vi "ABB Test Bearing run.vi"() -> ()   [LabVIEW 2017]
uses:
  Temp error msg.ctl
  Video Display Buttons.ctl
  ABB global.vi
panel:
  in  "Video Displays":T1
  in  "Temp error":T2="Error: Temperature measurement "
  out "Primary coolant":u16(ring) items=["Oil", "Water", "Natural"]
  in  "Start":bool
  out "Additional Temperatures":string[][](table)
  in  "Stabilitymessg":string="Thermal Stability reached"
  out "Time to Next reading":dbl(slide) scale=0.0..2.0 scale format="%#.1f"
  out "Start Time":dbl
  out "Temperatures":string[][](table)
  out "Readings":string[][](table)
  out "saved Readings":dbl[][](array[numeric])
  out "Serial number":string
  out "W.O number":string
  out "Norma 5000 Error":string
  in  "Record":bool
  out "Reading table":string[][](table)
  in  "View":enum16{"Graph", "Readings"}(ring)
  out "Number readings":i32
  out "Status":enum16{"Stopped", "Running", "Finished"}(ring)
  out "Timedate":string
  in  "End test":bool
  in  "Read Mode":enum16{"Auto", "Manual"}(ring)
  in  "Exit":bool
  out "Temperature Trend":cluster{dbl[], "Best Linear Fit":dbl[]}[](graph)
  # "Bearing Run"
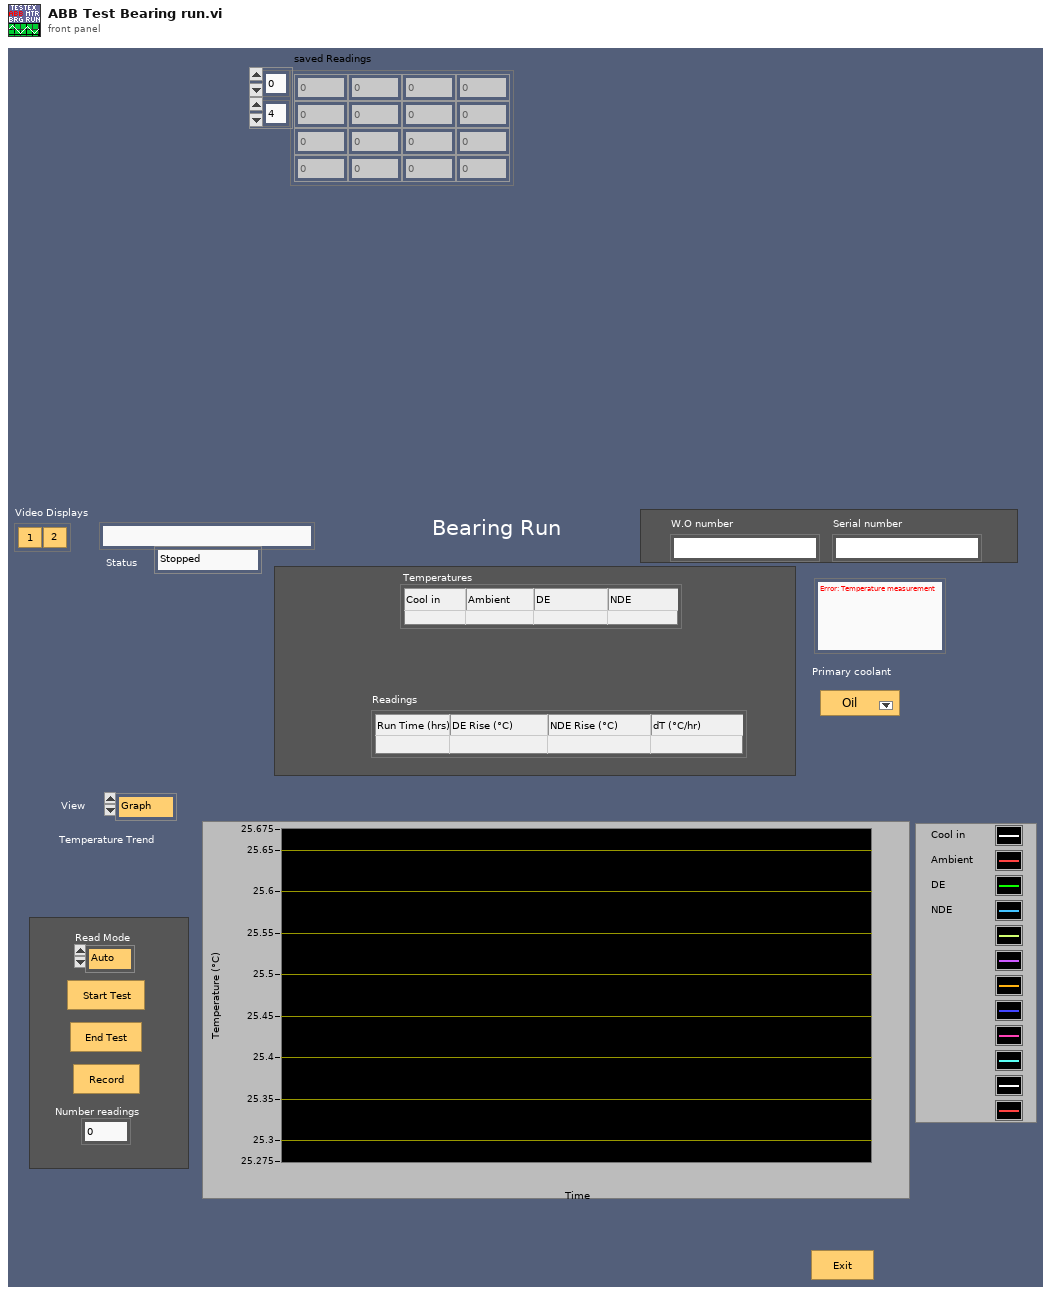
[diagram p1: front panel]
types:
  T1 = typedef "Video Display Buttons.ctl" = cluster{"1":bool, "1 2":bool}
  T2 = typedef "Temp error msg.ctl" = string
  T3 = enum16{"None", "Cool in", "Cool Out", "Wdg Temp", "Ambient", "DE", "NDE", "Aux coolant"}
  T4 = cluster{"VT Primary":dbl, "VT Secondary":dbl, "CT  Primary":dbl, "CT Secondary":dbl, "Current Shunt":enum16{"Internal", "External"}, "Avg interval":dbl}
  T5 = cluster{"VT Primary":dbl, "VT Secondary":dbl, "CT  Primary":dbl, "CT Secondary":dbl, "Current Shunt":enum16{"Internal", "External"}, "Averaging interval (secs)":dbl}
  T6 = cluster{"Visa sesssion":refnum<visa-resource-name>, "error":errorcluster}
  T7 = cluster{"Simulate Norma":bool, "Norma 5000 Address":u8, "WebDaq IP Address":string, "Simulate cDAQ":bool}
  T8 = cluster{"Thermal Stability (%)":dbl, "Reading interval (mins)":dbl}
  T9 = cluster{"String":string, "String":string, "String":string, "String":string}
  T10 = cluster{"String":dbl, "String":dbl, "String":dbl, "String":dbl}
  T11 = cluster{"temp. alloc":i32[], "category":i32[], "Category names":string[], "Category none names":string[]}
  T12 = cluster{"V":dbl, "A":dbl, "W":dbl, "VA":dbl, "VAr":dbl, "Pf":dbl}
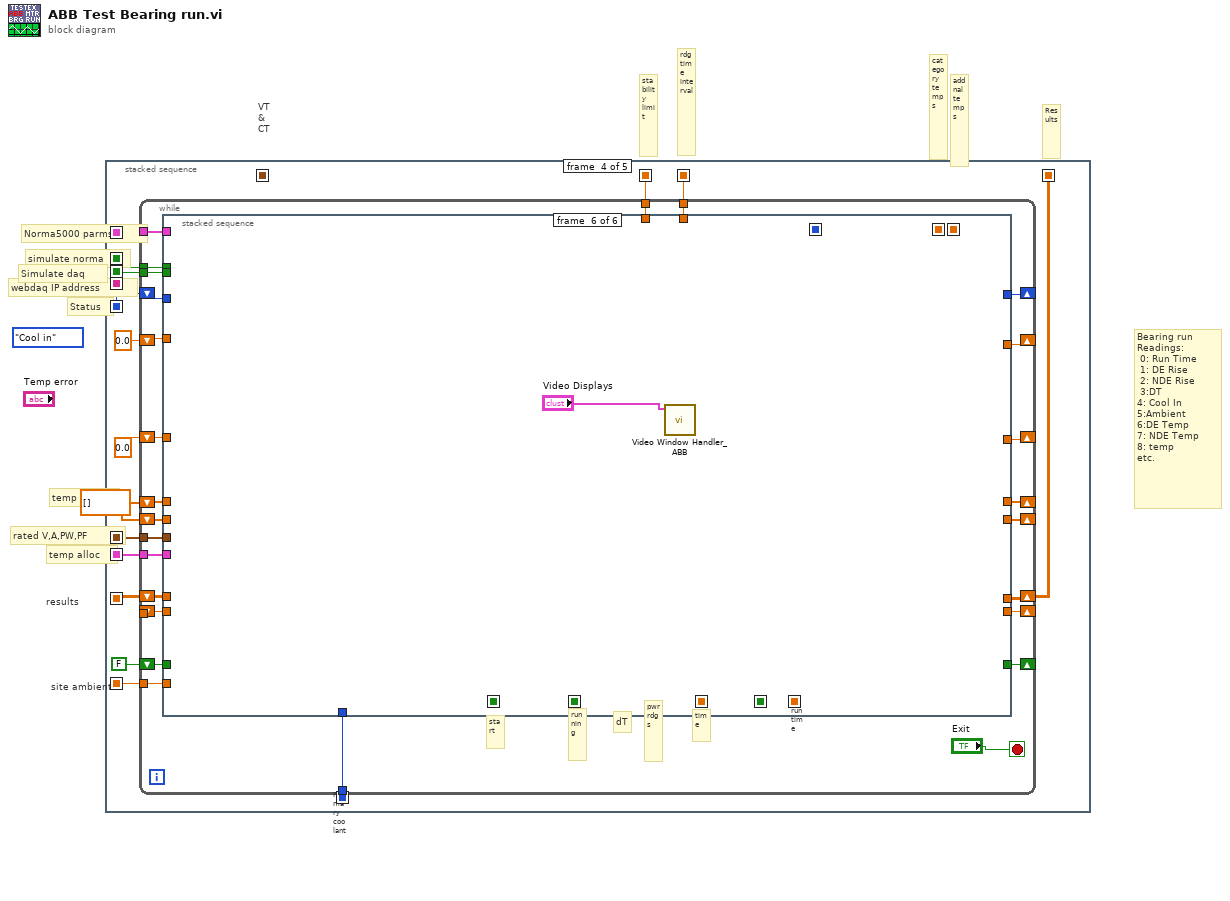
[diagram p0: block diagram]
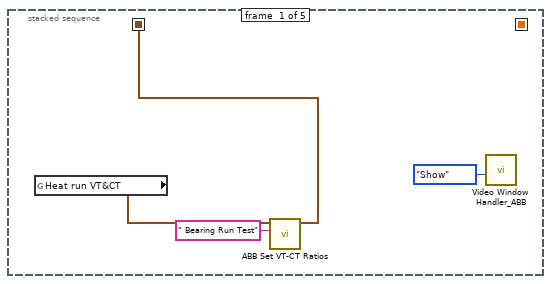
[diagram p2: hidden frame]
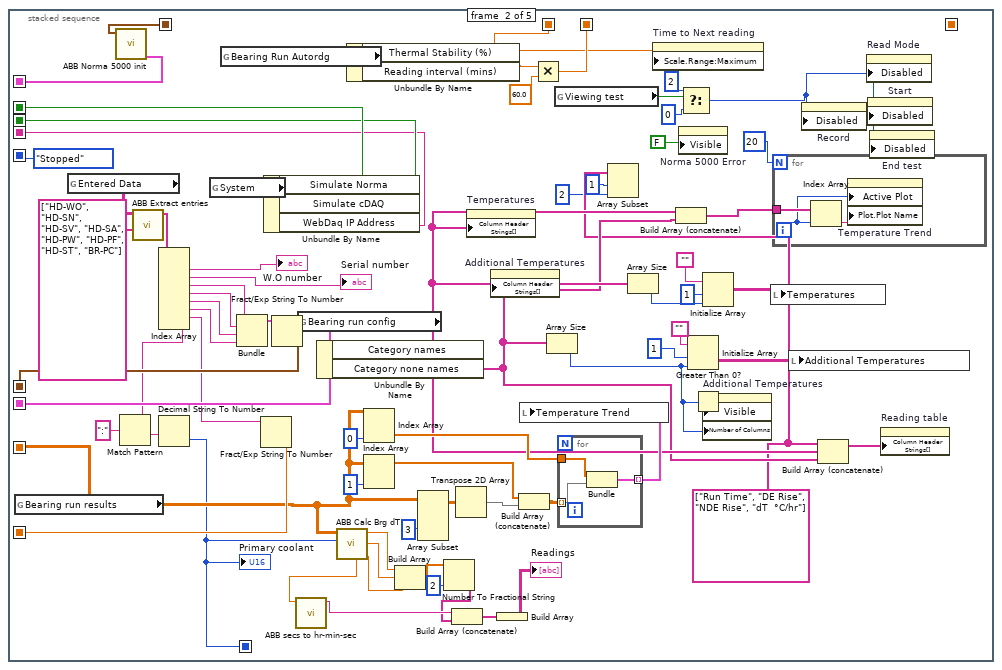
[diagram p3: hidden frame]
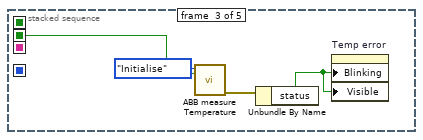
[diagram p4: hidden frame]
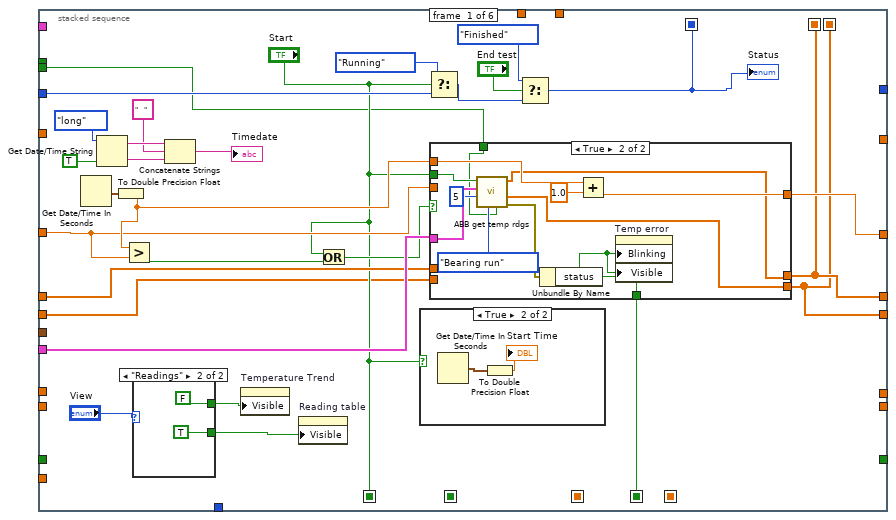
[diagram p5: hidden frame]
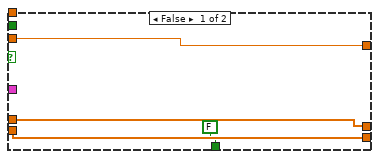
[diagram p7: hidden frame]
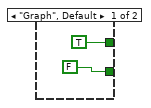
[diagram p8: hidden frame]
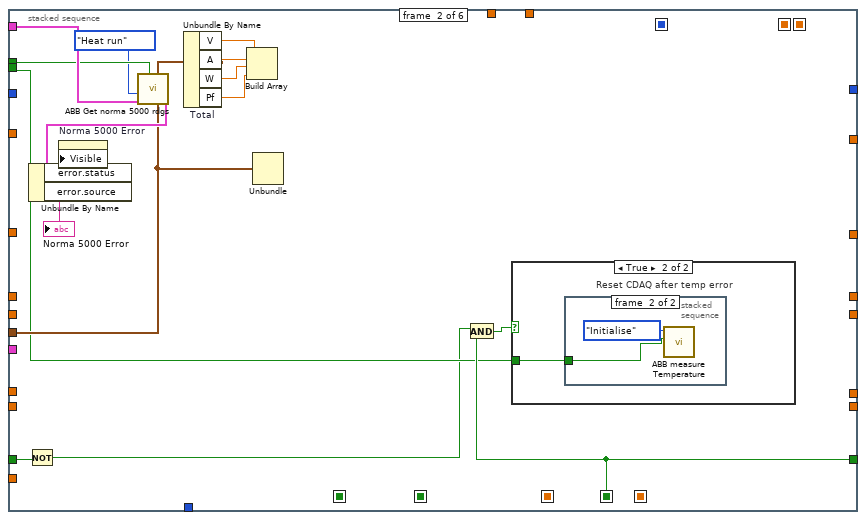
[diagram p9: hidden frame]
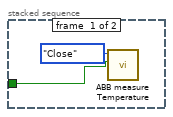
[diagram p11: hidden frame]
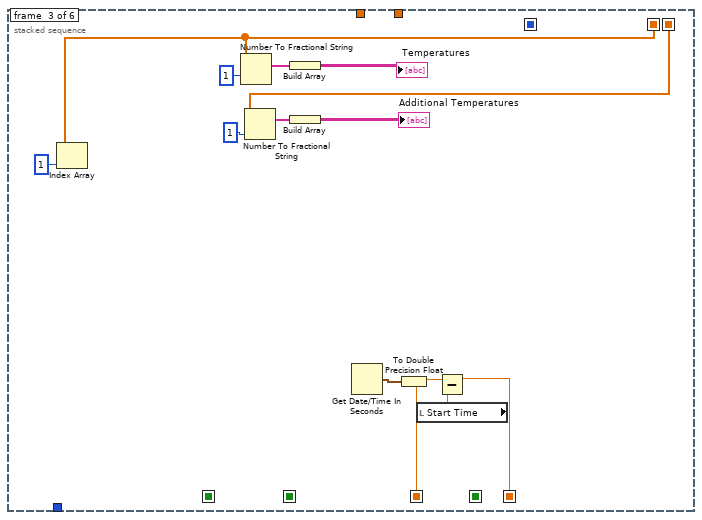
[diagram p12: hidden frame]
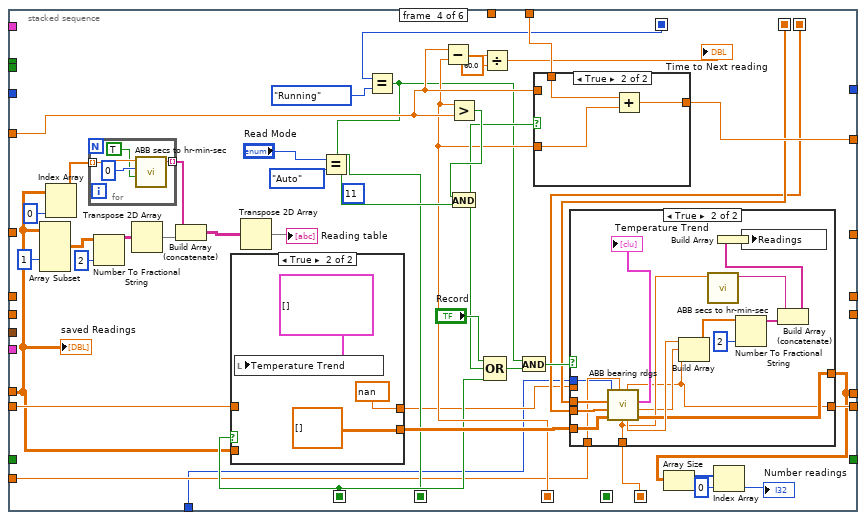
[diagram p13: hidden frame]
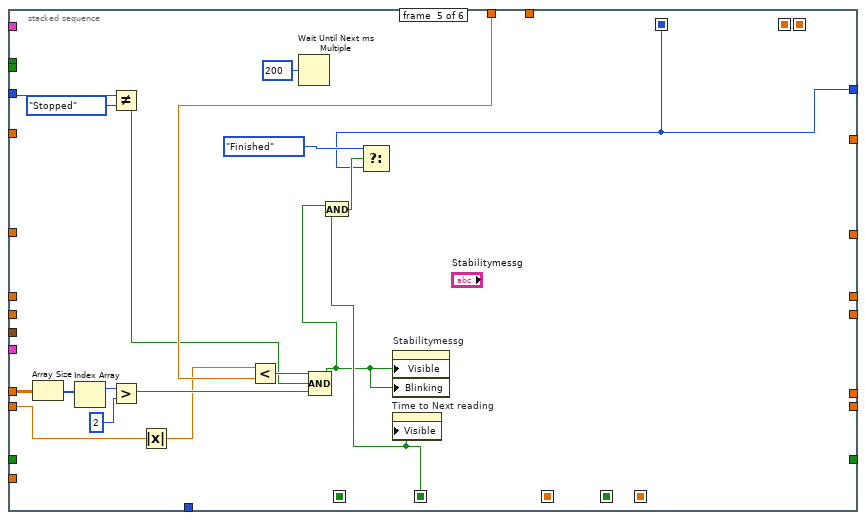
[diagram p17: hidden frame]
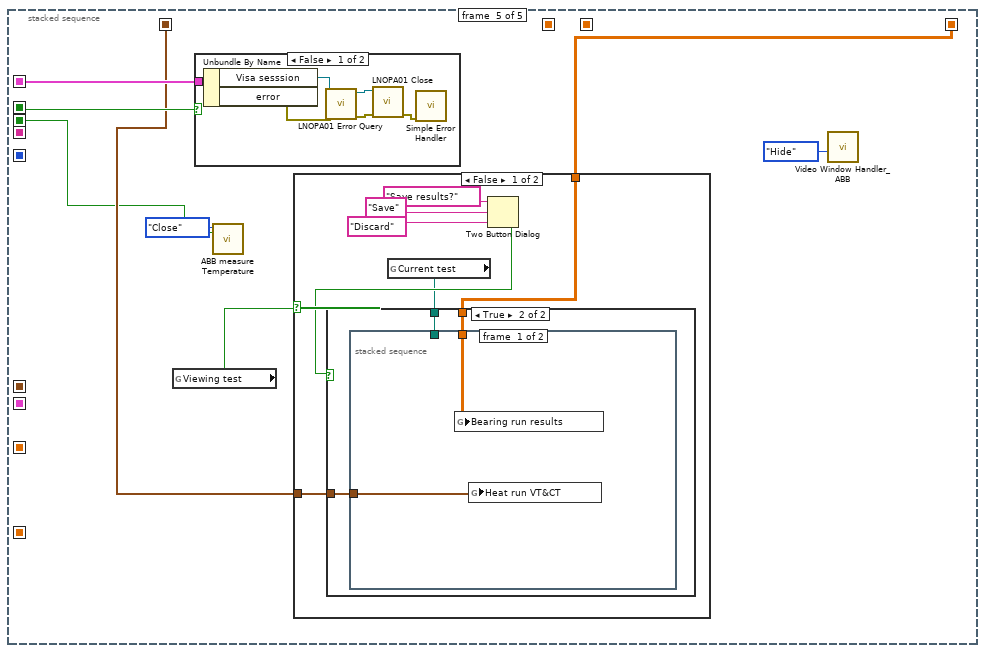
[diagram p18: hidden frame]
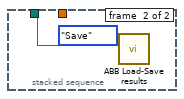
[diagram p20: hidden frame]
diagram:
  (unwired) T3."Cool in" ("Reading Category")
  # "Primary coolant"
  # "site ambient"
  # "results"
  # "VT & CT"
  # "webdaq IP address"
  # "Simulate daq"
  # "addnal temps"
  # "category temps"
  # "stability limit"
  # "Results"
  # "rdg time interval"
  # "Bearing run Readings:\n 0: Run Time\n 1: DE Rise\n 2: NDE Rise\n 3:DT\n4: Cool In\n5:Ambient\n6:DE Temp\n7: NDE Temp\n8: temp\netc."
  # "temp rdgs"
  # "temp alloc"
  # "rated V,A,PW,PF"
  # "simulate norma"
  # "Norma5000 parms"
  # "Status"
  n1 = stacked-sequence {
    seq-local: [_ enum16{"Stopped", "Running", "Finished"}."Stopped" ("Status") _ _ _] -> [_ _ _ w102 _]
    seq-local: [_ w75 _ _ _] -> [_ _ _ w101 w316]
    seq-local: [_ w72 _ _ _] -> [_ _ _ w100 w315]
    seq-local: [_ w71 _ _ _] -> [_ _ _ w99 _]
    seq-local: [_ w19 _ _ _] -> [_ _ _ w98 _]
    seq-local: [_ w35 _ _ _] -> [_ _ _ w97 _]
    seq-local: [_ w58 _ _ _] -> [_ _ _ w96 _]
    seq-local: [_ _ _ w94 _] -> [_ _ _ _ w313]
    seq-local: [_ w48 _ _ _] -> [_ _ _ w93 _]
    seq-local: [_ w32 _ _ _] -> [_ _ w86 w90 w310]
    seq-local: [_ w31 _ _ _] -> [_ _ _ _ _]
    seq-local: [w2 _ _ _ _] -> [_ w25 _ _ w312]
    seq-local: [_ w23 _ _ _] -> [_ _ _ w89 _]
    seq-local: [_ w18 _ _ _] -> [_ _ _ w88 _]
    frame #0 {
      n2 = global read "ABB global.vi" "Heat run VT&CT"() -> (w3:T4)
      n3 = call "ABB Set VT-CT Ratios.vi"("Test name"=" Bearing Run Test", "VT and CT Ratios"=w3) -> ("VT and CT Ratios out"=w2:T5)  [unwired: 9 in]
      n4 = call "Video Window Handler_ABB.vi"("Action"=enum16{"Show", "Hide", "Exit"}."Show") -> ()  [unwired: 11 in]
    }
    frame #1 {
      w7 = string[] ["Run Time", "DE Rise", "NDE Rise", "dT  °C/hr"]
      n5 = global read "ABB global.vi" "Bearing run results"() -> (w19:dbl[][])
      n6 = global read "ABB global.vi" "Entered Data"() -> (w55:string[][])
      n7 = call "ABB Norma 5000 init.vi"("VT and CT Ratios"=w25) -> ("norma 5000 parms out"=w75:T6)  [unwired: 10 in]
      n8 = call "ABB Extract entries.vi"("Entry IDs"=string[] ["HD-WO", "HD-SN", "HD-SV", "HD-SA", "HD-PW", "HD-PF", "HD-ST", "BR-PC"], "Entry table in"=w55) -> ("Selected Entries"=w53:string[])  [unwired: 9 in]
      n9 = Index Array(array=w53) -> (element #1=→"W.O number":string, element #2=→"Serial number":string, element #3=w50:string, element #4=w37:string, element #5=w36:string, element #6=w38:string, element #7=w24:string, element #8=w22:string)  [unwired: 8 in]
      n10 = Match Pattern(string=w22, regular expression=":") -> (after substring=w20:string)  [unwired: 1 in, 3 out]
      n11 = Decimal String To Number(string=w20) -> (number=w18:i32)  [unwired: 2 in, 1 out]
      "Primary coolant" <- w18
      n12 = global read "ABB global.vi" "System"() -> (w74:T7)
      n13 = global read "ABB global.vi" "Bearing Run Autordg"() -> (w70:T8)
      n14 = Bundle("String"=w50, "String"=w37, "String"=w36, "String"=w38) -> (w49:T9)  [unwired: 1 in]
      n15 = Fract/Exp String To Number(string=w24) -> (number=w23:dbl)  [unwired: 3 in, 1 out]
      n16 = Unbundle By Name(w74) -> ("Simulate Norma"=w72:bool, "Simulate cDAQ"=w32:bool, "WebDaq IP Address"=w31:string)
      n17 = Fract/Exp String To Number(string=w49) -> (number=w71:T10)  [unwired: 3 in, 1 out]
      n18 = global read "ABB global.vi" "Bearing run config"() -> (w35:T11)
      n19 = Unbundle By Name(w35) -> ("Category names"=w34:string[], "Category none names"=w29:string[])
      n20 = call "ABB Calc Brg dT.vi"("Primary coolant"=w18, "Readings in"=w19) -> ("dT (deg/hr)"=w13:dbl, "NDE rise"=w14:dbl, "DE rise"=w15:dbl, "run time"=w17:dbl)  [unwired: 5 in, 1 out]
      n21 = call "ABB secs to hr-min-sec.vi"("Seconds"=w17) -> ("hr:min:secs"=w16:string)  [unwired: 10 in]
      n22 = Unbundle By Name(w70) -> ("Thermal Stability (%)"=w48:dbl, "Reading interval (mins)"=w57:dbl)
      n23 = Index Array(array=w19, index (col)=0 ("disabled index (col)")) -> (element=w63:dbl[])  [unwired: 1 in]
      n24 = Index Array(array=w19, index (col)=1 ("disabled index (col)")) -> (element=w26:dbl[])  [unwired: 1 in]
      n25 = Build Array(w15, w14, w13) -> (w12:dbl[])
      n26 = Array Subset(array=w19, index (col)=3 ("index")) -> (w61:dbl[][])  [unwired: 3 in]
      n27 = Number To Fractional String(number=w12, precision (6)=i16 2) -> (F-format string=w10:string[])  [unwired: 2 in]
      n28 = Build Array (concatenate)(w16, w10) -> (w9:string[])
      n29 = Transpose 2D Array(2D array=w61) -> (transposed array=w60:dbl[][])
      n30 = property on="Temperatures" class="Tbl (strict)"("Column Header Strings[]"=w34) -> ()  [unwired: 2 in, 2 out]
      n31 = property on="Additional Temperatures" class="Tbl (strict)"("Column Header Strings[]"=w29) -> ()  [unwired: 2 in, 2 out]
      n32 = Build Array(w9) -> (→"Readings":string[][])
      n33 = Build Array (concatenate)(w26, w60) -> (w27:dbl[][])
      n34 = Multiply(x=w57, y=60.0) -> (x*y=w58:dbl)
      n35 = Array Size(array=w29) -> (size(s)=w33:i32)
      n36 = global read "ABB global.vi" "Viewing test"() -> (w42:bool)
      n37 = for {
        tunnel: w63 -> [w79]
        tunnel: w27 -> [w78] mode=indexing
        tunnel: [w77] -> w59 mode=indexing
        n38 = Bundle("Bearing run results"=w79, w78) -> (w77:cluster{"Bearing run results":dbl[], dbl[]})  [unwired: 1 in]
      }
      n39 = local write "Temperature Trend"(w59) -> ()
      n40 = Array Subset(array=w7, index=1, length=2) -> ()  [unwired: 1 out]
      n41 = Array Size(array=w34) -> (size(s)=w68:i32)
      n42 = property on="Time to Next reading" class="Slide (strict)"("Scale.Range:Maximum"=w57) -> ()  [unwired: 2 in, 2 out]
      n43 = Build Array (concatenate)(w34, w29) -> (w30:string[])
      n44 = property on="Norma 5000 Error" class="Str"("Visible"=FALSE) -> ()  [unwired: 2 in, 2 out]
      n45 = Select(t=2, s=w42, f=0) -> (s? t:f=w39:i32)
      n46 = Initialize Array("", 1 ("dimension size"), w33) -> (w45:string[][])
      n47 = Greater Than 0?(x=w33) -> (x > 0?=w44:bool)
      n48 = Initialize Array("", 1 ("dimension size"), w68) -> (w66:string[][])
      n49 = property on="Additional Temperatures" class="Tbl (strict)"("Visible"=w44, "Number of Columns"=w33) -> ()  [unwired: 2 in, 2 out]
      n50 = local write "Temperatures"(w66) -> ()
      n51 = for {
        N: 20 -> [_]
        tunnel: w30 -> [w82]
        i -> [w81]
        n52 = Index Array(array=w82, index=w81) -> (element=w80:string)
        n53 = property on="Temperature Trend" class="XYGraph (strict)"("Active Plot"=w81, "Plot.Plot Name"=w80) -> ()  [unwired: 2 in, 2 out]
      }
      n54 = local write "Additional Temperatures"(w45) -> ()
      n55 = property on="Record" class="Bool"("Disabled"=w39) -> ()  [unwired: 2 in, 2 out]
      n56 = Build Array (concatenate)(w7, w34, w29) -> (w56:string[])
      n57 = property on="Read Mode" class="Enum (strict)"("Disabled"=w39) -> ()  [unwired: 2 in, 2 out]
      n58 = property on="Start" class="Bool"("Disabled"=w39) -> ()  [unwired: 2 in, 2 out]
      n59 = property on="End test" class="Bool"("Disabled"=w39) -> ()  [unwired: 2 in, 2 out]
      n60 = property on="Reading table" class="Tbl (strict)"("Column Header Strings[]"=w56) -> ()  [unwired: 2 in, 2 out]
    }
    frame #2 {
      n61 = call "ABB measure Temperature.vi"("Simulate"=w86, "Mode"=enum16{"Initialise", "Read", "Close"}."Initialise") -> ("error out"=w84:errorcluster)  [unwired: 7 in, 2 out]
      n62 = Unbundle By Name(w84) -> ("status"=w83:bool)
      n63 = property on="Temp error" class="Str (strict)"("Blinking"=w83, "Visible"=w83) -> ()  [unwired: 2 in, 2 out]
    }
    frame #3 {
      w92 = dbl[] []
      n64 = while {
        shift-right: [w126] -> _
        shift-left: w102 -> [w127]
        tunnel: w101 -> [w125]
        tunnel: w100 -> [w124]
        tunnel: w99 -> [w123]
        shift-right: [w121] -> w94
        shift-left: w98 -> [w122]
        shift-right: [w118] -> _
        shift-left: 0.0 -> [w120]
        shift-right: [w119] -> _
        shift-left: w92 -> [w116]
        tunnel: w97 -> [w117]
        tunnel: w96 -> [w115]
        shift-right: [w113] -> _
        shift-left: 0.0 -> [w114]
        tunnel: w93 -> [w112]
        shift-right: [w110] -> _
        shift-left: w92 -> [w111]
        tunnel: w90 -> [w109]
        shift-right: [w108] -> _
        shift-left: _ -> [w107]
        tunnel: [w107] -> _
        tunnel: w89 -> [w106]
        tunnel: w88 -> [w105]
        shift-right: [w104] -> _
        shift-left: FALSE ("status") -> [w103]
        stop <- "Exit" stop-if-true
        # "run time"
        # "running"
        # "time"
        # "dT"
        # "pwr rdgs"
        # "start"
        n65 = stacked-sequence {
          seq-local: ["Start" _ _ _ _ _] -> [_ _ _ w241 _ _]
          seq-local: [_ _ w211 _ _ _] -> [_ _ _ w245 _ _]
          seq-local: [w135 _ _ _ _ _] -> [_ _ _ w239 w291 _]
          seq-local: [w134 _ _ _ _ _] -> [_ _ w203 w238 _ _]
          seq-local: [_ _ _ w237 _ _] -> [_ _ _ _ w296 _]
          seq-local: [w131 _ _ _ _ _] -> [_ _ w208 w236 _ _]
          seq-local: [_ _ w204 _ _ _] -> [_ _ _ w235 _ _]
          seq-local: [w129 _ _ _ _ _] -> [_ w183 _ _ _ _]
          tunnel: w127 -> [w151 _ _ _ w300 _]
          tunnel: [_ _ _ _ w291 _] -> w126
          tunnel: w125 -> [_ w196 _ _ _ _]
          tunnel: w124 -> [_ w192 _ _ _ _]
          tunnel: w123 -> [_ w189 _ _ _ _]
          tunnel: w122 -> [_ _ _ w224 w304 _]
          tunnel: [_ _ _ w219 _ _] -> w121
          tunnel: w120 -> [w141 _ _ _ _ _]
          tunnel: [w134 _ _ _ _ _] -> w119
          tunnel: [w140 _ _ _ _ _] -> w118
          tunnel: w117 -> [w139 _ _ _ _ _]
          tunnel: w116 -> [w138 _ _ _ _ _]
          tunnel: w115 -> [_ _ _ w256 _ _]
          tunnel: w114 -> [_ _ _ w246 _ _]
          tunnel: [_ _ _ w255 _ _] -> w113
          tunnel: w112 -> [_ _ _ _ w303 _]
          tunnel: w111 -> [w132 _ _ _ _ _]
          tunnel: [w131 _ _ _ _ _] -> w110
          tunnel: w109 -> [w130 w182 _ _ _ _]
          tunnel: [_ _ _ w234 _ _] -> w108
          tunnel: w107 -> [_ _ _ w233 w292 _]
          tunnel: w106 -> [_ _ _ w216 _ _]
          tunnel: w105 -> [_ _ _ w215 _ _]
          tunnel: [_ w183 _ _ _ _] -> w104
          tunnel: w103 -> [_ w181 _ _ _ _]
          frame #0 {
            n66 = Get Date/Time In Seconds() -> (seconds since 1Jan1904=w143:timestamp)
            n67 = Get Date/Time String(date format (0)=enum16{"short", "long", "abbreviated"}."long", want seconds? (F)=TRUE) -> (date string=w155:string, time string=w154:string)  [unwired: 1 in]
            n68 = To Double Precision Float(number=w143) -> (double precision float=w142:dbl)
            n69 = Greater?(x=w142, y=w141) -> (0:w137:bool)
            n70 = case shown="\"Readings\"" "View" {
              tunnel: [TRUE FALSE] -> w145
              tunnel: [FALSE TRUE] -> w144
              frame "Graph", Default {
              }
              frame "Readings" {
              }
            }
            n71 = Concatenate Strings(w155, "   ", w154) -> (→"Timedate":string)
            n72 = property on="Temperature Trend" class="XYGraph (strict)"("Visible"=w145) -> ()  [unwired: 2 in, 2 out]
            n73 = property on="Reading table" class="Tbl (strict)"("Visible"=w144) -> ()  [unwired: 2 in, 2 out]
            n74 = Or(x="Start", y=w137) -> (x .or. y?=w136:bool)
            n75 = case shown="True" "Start" {
              frame False {
              }
              frame True {
                n76 = Get Date/Time In Seconds() -> (seconds since 1Jan1904=w159:timestamp)
                n77 = To Double Precision Float(number=w159) -> (double precision float=→"Start Time":dbl)
              }
            }
            n78 = Select(t=enum16{"Stopped", "Running", "Finished"}."Running", s="Start", f=w151) -> (s? t:f=w149:enum16{"Stopped", "Running", "Finished"})
            n79 = case shown="True" w136 {
              tunnel: w142 -> [_ w175]
              tunnel: [w163 w173] -> w140
              tunnel: w141 -> [w163 _]
              tunnel: w130 -> [_ w166]
              tunnel: w139 -> [_ w171]
              tunnel: [w162 w170] -> w134
              tunnel: w138 -> [w162 _]
              tunnel: "Start" -> [_ w172]
              tunnel: w132 -> [w161 _]
              tunnel: [w161 w169] -> w131
              tunnel: [FALSE ("status") w164] -> w129
              frame False {
              }
              frame True {
                n80 = call "ABB get temp rdgs.vi"("Sim daq"=w166, "sim type"=enum16{"Heat run", "Bearing run"}."Bearing run", "# categories"=5, "run config"=w171, "start"=w172) -> ("error out"=w165:errorcluster, "Category none rdgs"=w169:dbl[], "Category rdgs"=w170:dbl[])  [unwired: 3 in, 1 out]
                n81 = Unbundle By Name(w165) -> ("status"=w164:bool)
                n82 = Add(x=w175, y=1.0) -> (x+y=w173:dbl)
                n83 = property on="Temp error" class="Str (strict)"("Blinking"=w164, "Visible"=w164) -> ()  [unwired: 2 in, 2 out]
              }
            }
            n84 = Select(t=enum16{"Stopped", "Running", "Finished"}."Finished", s="End test", f=w149) -> (s? t:f=w135:enum16{"Stopped", "Running", "Finished"})
            "Status" <- w135
          }
          frame #1 {
            n85 = Not(x=w181) -> (.not. x?=w180:bool)
            n86 = call "ABB Get norma 5000 rdgs.vi"("Rated"=w189, "simulate"=w192, "norma 5000 parms in"=w196, "Simulate Mode"=enum16{"No load", "Locked Rotor", "Heat run"}."Heat run") -> ("norma 5000 parms out"=w193:T6, "Total"=w190:T12)  [unwired: 3 in, 3 out]
            n87 = Unbundle By Name(w193) -> ("error.status"=w195:bool, "error.source"=→"Norma 5000 Error":string)
            n88 = property on="Norma 5000 Error" class="Str"("Visible"=w195) -> ()  [unwired: 2 in, 2 out]
            n89 = Unbundle By Name "Total"(w190) -> ("V"=w188:dbl, "A"=w187:dbl, "W"=w186:dbl, "Pf"=w185:dbl)
            n90 = Build Array(w188, w187, w186, w185) -> ()  [unwired: 1 out]
            n91 = Unbundle(w189) -> ()  [unwired: 4 out]
            n92 = And(x=w180, y=w183) -> (x .and. y?=w184:bool)
            n93 = case shown="True" w184 {
              tunnel: w182 -> [_ w197]
              frame False {
              }
              frame True {
                # "Reset CDAQ after temp error"
                n94 = stacked-sequence {
                  tunnel: w197 -> [w198 w200]
                  frame #0 {
                    n95 = call "ABB measure Temperature.vi"("Simulate"=w198, "Mode"=enum16{"Initialise", "Read", "Close"}."Close") -> ()  [unwired: 7 in, 3 out]
                  }
                  frame #1 {
                    n96 = call "ABB measure Temperature.vi"("Simulate"=w200, "Mode"=enum16{"Initialise", "Read", "Close"}."Initialise") -> ()  [unwired: 7 in, 3 out]
                  }
                }
              }
            }
          }
          frame #2 {
            n97 = Index Array(array=w203, index=1) -> ()  [unwired: 1 out]
            n98 = Number To Fractional String(number=w203, precision (6)=i16 1) -> (F-format string=w209:string[])  [unwired: 2 in]
            n99 = Number To Fractional String(number=w208, precision (6)=i16 1) -> (F-format string=w207:string[])  [unwired: 2 in]
            n100 = Build Array(w209) -> (→"Temperatures":string[][])
            n101 = Build Array(w207) -> (→"Additional Temperatures":string[][])
            n102 = Get Date/Time In Seconds() -> (seconds since 1Jan1904=w213:timestamp)
            n103 = To Double Precision Float(number=w213) -> (double precision float=w211:dbl)
            n104 = local read "Start Time"() -> (w212:dbl)
            n105 = Subtract(x=w211, y=w212) -> (x-y=w204:dbl)
          }
          frame #3 {
            (unwired) 11 ("index")
            n106 = Array Subset(array=w224, index (col)=1 ("index")) -> (w229:dbl[][])  [unwired: 3 in]
            n107 = Index Array(array=w224, index (col)=0 ("disabled index (col)")) -> (element=w228:dbl[])  [unwired: 1 in]
            n108 = for {
              tunnel: w228 -> [w261] mode=indexing
              tunnel: [w259] -> w226 mode=indexing
              n109 = call "ABB secs to hr-min-sec.vi"("round off secs"=TRUE, "Precision"=i16 0, "Seconds"=w261) -> ("hr:min:secs"=w259:string)  [unwired: 8 in]
            }
            n110 = Number To Fractional String(number=w229, precision (6)=i16 2) -> (F-format string=w230:string[][])  [unwired: 2 in]
            n111 = Transpose 2D Array(2D array=w230) -> (transposed array=w225:string[][])
            n112 = Build Array (concatenate)(w226, w225) -> (w227:string[][])
            n113 = case shown="True" w241 {
              tunnel: w224 -> [w267 _]
              tunnel: [w267 dbl[][] []] -> w249
              tunnel: w233 -> [w266 _]
              tunnel: [w266 nan] -> w232
              frame False {
              }
              frame True {
                n114 = local write "Temperature Trend"(cluster{dbl[], "Best Linear Fit":dbl[]}[] [] ("Temperature Trend")) -> ()
              }
            }
            n115 = Transpose 2D Array(2D array=w227) -> (transposed array=→"Reading table":string[][])
            n116 = Equal?(x="Read Mode", y=enum16{"Auto", "Manual"}."Auto") -> (x = y?=w252:bool)
            n117 = Equal?(x=w239, y=enum16{"Stopped", "Running", "Finished"}."Running" ("x")) -> (x = y?=w237:bool)
            n118 = Subtract(x=w246, y=w245) -> (x-y=w244:dbl)
            n119 = Greater?(x=w245, y=w246) -> (0:w251:bool)
            n120 = And(x=w251, y=w252) -> (x .and. y?=w250:bool)
            n121 = Divide(x=w244, y=60.0) -> (x/y=→"Time to Next reading":dbl)
            n122 = Compound Arithmetic op=OR("Record", w250, w241) -> (w247:bool)
            n123 = And(x=w237, y=w247) -> (x .and. y?=w248:bool)
            n124 = case shown="True" w250 {
              tunnel: w256 -> [_ w264]
              tunnel: w245 -> [_ w265]
              tunnel: [w262 w263] -> w255
              tunnel: w246 -> [w262 _]
              frame False {
              }
              frame True {
                n125 = Add(x=w264, y=w265) -> (x+y=w263:dbl)
              }
            }
            n126 = case shown="True" w248 {
              tunnel: w249 -> [w272 w282]
              tunnel: [w272 w281] -> w219
              tunnel: w238 -> [_ w280]
              tunnel: w236 -> [_ w279]
              tunnel: w235 -> [_ w278]
              tunnel: [w271 w273] -> w234
              tunnel: w232 -> [w271 _]
              tunnel: w216 -> [_ w276]
              tunnel: w215 -> [_ w275]
              frame False {
              }
              frame True {
                n127 = call "ABB bearing rdgs.vi"("Run Time"=w278, "Site ambient"=w276, "Readings in"=w282, "Aditional temps"=w279, "temperatures"=w280, "Primary coolant"=w275) -> ("Readings out"=w281:dbl[][], "NDE rise"=w274:dbl, "Temperature trend"=→"Temperature Trend":cluster{dbl[], dbl[]}[], "DE rise"=w284:dbl, "rise rate"=w273:dbl)  [unwired: 1 in]
                n128 = Build Array(w284, w274, w273) -> (w287:dbl[])
                n129 = call "ABB secs to hr-min-sec.vi"("Seconds"=w278) -> ("hr:min:secs"=w285:string)  [unwired: 10 in]
                n130 = Number To Fractional String(number=w287, precision (6)=i16 2) -> (F-format string=w289:string[])  [unwired: 2 in]
                n131 = Build Array (concatenate)(w285, w289) -> (w288:string[])
                n132 = Build Array(w288) -> (w277:string[][])
                n133 = local write "Readings"(w277) -> ()
              }
            }
            n134 = Array Size(array=w219) -> (size(s)=w220:i32[])
            n135 = Index Array(array=w220, index=0) -> (element=→"Number readings":i32)
            "saved Readings" <- w224
          }
          frame #4 {
            n136 = Array Size(array=w304) -> (size(s)=w307:i32[])
            n137 = Index Array(array=w307) -> (element=w306:i32)  [unwired: 1 in]
            n138 = Not Equal?(x=w300, y=enum16{"Stopped", "Running", "Finished"}."Stopped") -> (x != y?=w298:bool)
            n139 = Greater?(x=w306, y=2) -> (0:w301:bool)
            n140 = Absolute Value(x=w292) -> (abs(x)=w290:dbl)
            n141 = Less?(x=w290, y=w303) -> (x < y?=w302:bool)
            n142 = Wait Until Next ms Multiple(millisecond multiple=u32 200) -> ()  [unwired: 1 out]
            n143 = Compound Arithmetic op=AND(w302, w298, w301) -> (w295:bool)
            n144 = And(x=w295, y=w296) -> (x .and. y?=w294:bool)
            n145 = Select(t=enum16{"Stopped", "Running", "Finished"}."Finished", s=w294, f=w291) -> ()  [unwired: 1 out]
            n146 = property on="Stabilitymessg" class="Str"("Visible"=w295, "Blinking"=w295) -> ()  [unwired: 2 in, 2 out]
            n147 = property on="Time to Next reading" class="Slide (strict)"("Visible"=w296) -> ()  [unwired: 2 in, 2 out]
          }
          frame #5 {
            n148 = call "Video Window Handler_ABB.vi"("Video Displays"="Video Displays") -> ()  [unwired: 11 in]
          }
        }
      }
    }
    frame #4 {
      n149 = global read "ABB global.vi" "Viewing test"() -> (w314:bool)
      n150 = case shown="False" w315 {
        tunnel: w316 -> [w333 _]
        frame False {
          n151 = Unbundle By Name(w333) -> ("Visa sesssion"=w332:refnum<visa-resource-name>, "error"=w331:errorcluster)
          n152 = call "LNOPA01 Error Query.vi"("error in (no error)"=w331, "VISA session"=w332) -> ("error out"=w334:errorcluster, "dup VISA session"=w335:refnum<visa-resource-name>)  [unwired: 6 in, 2 out]
          n153 = call "LNOPA01 Close.vi"("error in (no error)"=w334, "VISA session"=w335) -> ("error out"=w336:errorcluster)  [unwired: 9 in]
          n154 = call <vilib>:"Simple Error Handler.vi"("error in (no error)"=w336) -> ()  [unwired: 4 in, 5 out]
        }
        frame True {
        }
      }
      n155 = call "ABB measure Temperature.vi"("Simulate"=w310, "Mode"=enum16{"Initialise", "Read", "Close"}."Close") -> ()  [unwired: 7 in, 3 out]
      n156 = case shown="False" w314 {
        tunnel: w313 -> [w321 _]
        tunnel: w312 -> [w317 _]
        frame False {
          n157 = global read "ABB global.vi" "Current test"() -> (w320:path)
          n158 = Two Button Dialog(message="Save results?", 1:"Discard" ("F button name (\"Cancel\")"), 2:"Save" ("T button name (\"OK\")")) -> (T button?=w322:bool)
          n159 = case shown="True" w322 {
            tunnel: w321 -> [_ w326]
            tunnel: w320 -> [_ w325]
            tunnel: w317 -> [_ w324]
            frame False {
            }
            frame True {
              n160 = stacked-sequence {
                tunnel: w326 -> [w328 _]
                tunnel: w325 -> [_ w329]
                tunnel: w324 -> [w327 _]
                frame #0 {
                  n161 = global write "ABB global.vi" "Bearing run results"(w328) -> ()
                  n162 = global write "ABB global.vi" "Heat run VT&CT"(w327) -> ()
                }
                frame #1 {
                  n163 = call "ABB Load-Save results.vi"("Path"=w329, "Mode"=enum16{"LOAD", "Save"}."Save") -> ()  [unwired: 10 in]
                }
              }
            }
          }
        }
        frame True {
        }
      }
      n164 = call "Video Window Handler_ABB.vi"("Action"=enum16{"Show", "Hide", "Exit"}."Hide") -> ()  [unwired: 11 in]
    }
  }
